vi "Get ClassID Name__ogtk.vi"(8 "error in (no error)":errorcluster, 11 "Gen Refnum":refnum<vi>) -> (0 "error out":errorcluster, 1 "ClassID Mapped?":bool, 2 "ClassID Name":T1=enum."Decoration", 3 "dup Gen Refnum":refnum<vi>)   [LabVIEW 2011]
doc: "Gets the ClassID of a LabVIEW object by RefNum and outputs an enumeration using names such as \"Digital Numeric\", \"Boolean\", \"String\", \"Path\", etc."
uses:
  ClassID Names Enum__ogtk.ctl
panel:
  # "Get ClassID Name.vi\n\nGets the ClassID of a LabVIEW object by RefNum and outputs an enumeration using names such as \"Digital Numeric\",  \"Boolean\", \"String\", \"Path\", etc.\n\nPlease visit http://www.OpenG.org to learn about the\nOpen Source LabVIEW software movement.\n\nNOTICE -- YOU MUST LEAVE THIS NOTICE IN PLACE.  PER THE TERMS OF THE LICENSE BELOW, YOU MAY SUBLICENSE THIS SOFTWARE \nIN ANY WAY THAT DOES NOT CONFLICT WITH THIS LICENSE.\n\n### BSD License (http://www.opensource.org/licenses/bsd-license.php) Begin ###\n \nCopyright (c) 2002, Jim Kring <jim@jimkring.com>\n\nAll rights reserved.\n\nRedistribution and use in source and binary forms, with or without modification, are permitted provided that the following conditions are met:\n\n    * Redistributions of source code must retain the above copyright notice, this list of conditions and the following disclaimer.\n    * Redistributions in binary form must reproduce the above copyright notice, this list of conditions and the following disclaimer in the \n       documentation and/or other materials provided with the distribution.\n    * Neither the name of SciWare, James Kring, Inc., nor the names of its contributors may be used to endorse or promote products derived \n       from this software without specific prior written permission.\n\nTHIS SOFTWARE IS PROVIDED BY THE COPYRIGHT HOLDERS AND CONTRIBUTORS \"AS IS\" AND ANY EXPRESS OR IMPLIED WARRANTIES, \nINCLUDING, BUT NOT LIMITED TO, THE IMPLIED WARRANTIES OF MERCHANTABILITY AND FITNESS FOR A PARTICULAR PURPOSE ARE \nDISCLAIMED. IN NO EVENT SHALL THE COPYRIGHT OWNER OR CONTRIBUTORS BE LIABLE FOR ANY DIRECT, INDIRECT, INCIDENTAL,\n SPECIAL, EXEMPLARY, OR CONSEQUENTIAL DAMAGES (INCLUDING, BUT NOT LIMITED TO, PROCUREMENT OF SUBSTITUTE GOODS OR \nSERVICES; LOSS OF USE, DATA, OR PROFITS; OR BUSINESS INTERRUPTION) HOWEVER CAUSED AND ON ANY THEORY OF LIABILITY, \nWHETHER IN CONTRACT, STRICT LIABILITY, OR TORT (INCLUDING NEGLIGENCE OR OTHERWISE) ARISING IN ANY WAY OUT OF THE USE \nOF THIS SOFTWARE, EVEN IF ADVISED OF THE POSSIBILITY OF SUCH DAMAGE.\n\n### BSD License End ###"
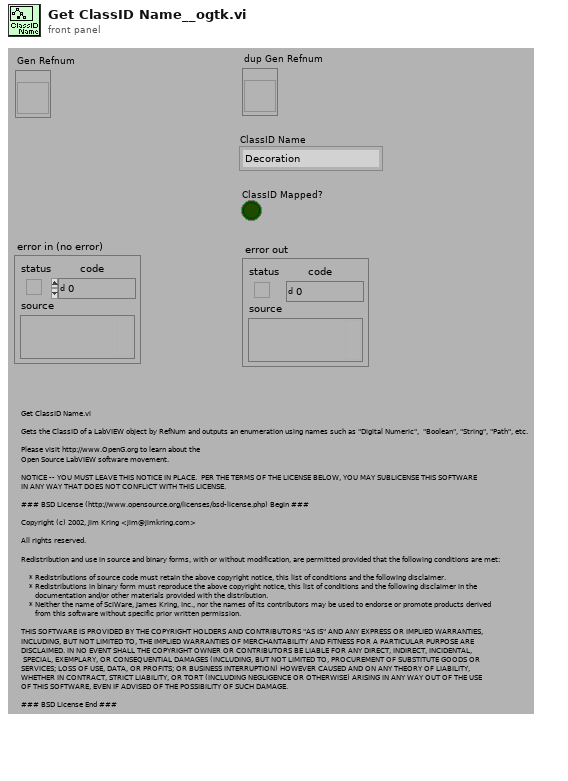
[diagram p1: front panel]
types:
  T1 = typedef "ClassID Names Enum__ogtk.ctl" = enum32{"0 <undefined>", "1 <undefined>", "2 <undefined>", "Generic", "Decoration", "Text", "Control", "ColorBox", "Boolean", "RefNum", "Variant", "Path", "ListBox", "Table", "Array", "Picture", "ActiveXContainer", "Numeric", "Digital", "NamedNumeric", "ColorRamp", "Slide", "GraphOrChart", "WaveformChart", "WaveformGraph", "IntensityChart", "IntensityGraph", "String", "IOName", "ComboBox", "Cluster", "Panel", "Knob", "NumWithScale", "Ring", "Enum", "GObject", "Plot", "Cursor", "NumericText", "Scale", "ColorScale", "GraphScale", "ColorGraphScale", "TypedRefNum", "OldKnobScale", "MCListbox", "MeasureData", "BVTag", "DAQName", "VISAName", "IVIName", "SlideScale", "TabControl", "Page", "TabArrayTabControl", "ConPane"}
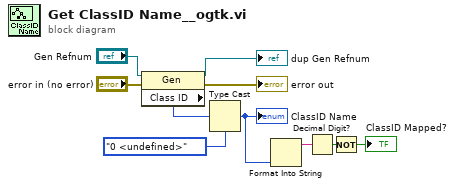
[diagram p0: block diagram]
diagram:
  n1 = property class="Gen"(reference="Gen Refnum", error in="error in (no error)") -> (reference out=→"dup Gen Refnum":refnum<vi>, error out=→"error out":errorcluster, "Class ID"=w6:u32)
  n2 = Type Cast(type=ClassID_Names_Enum__ogtk."0 <undefined>" ("ClassID Name"), x=w6) -> (*(type *) &x=w3:T1)
  "ClassID Name" <- w3
  n3 = Format Into String(w3) -> (resulting string=w5:string)  [unwired: 3 in, 1 out]
  n4 = Decimal Digit?(1:w5) -> (0:w4:bool)
  n5 = Not(x=w4) -> (.not. x?=→"ClassID Mapped?":bool)
